vi "Read Configuration.vi"(8 "error in (no error)":errorcluster, 11 "Measure Object in":refnum<class "da Base.lvclass">) -> (0 "error out":errorcluster, 2 "Configuration":variant, 3 "Measure Object out":refnum<class "da Base.lvclass">)   [LabVIEW 2016, in "da Base.lvclass"]
uses:
  da Base.lvclass
  da Base.lvclass/da Base.ctl
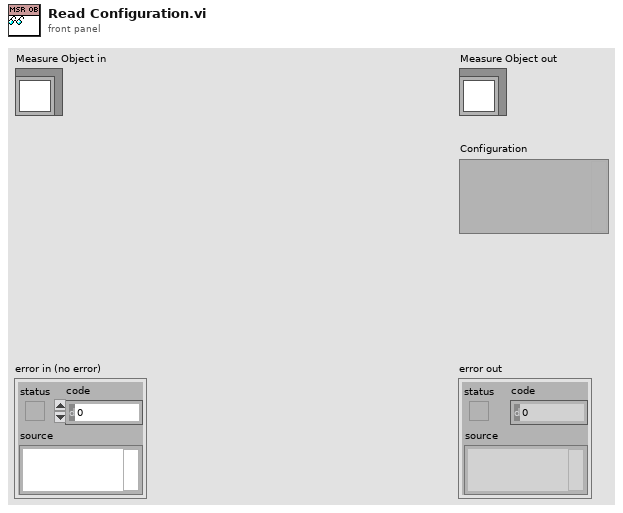
[diagram p1: front panel]
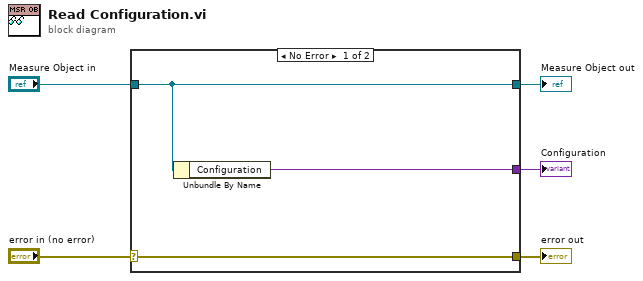
[diagram p0: block diagram]
diagram:
  n1 = case shown="No Error" "error in (no error)" {
    selector: "error in (no error)" -> [w8 w9]
    tunnel: [w8 w9] -> w4
    tunnel: [w7 w10] -> w2
    tunnel: "Measure Object in" -> [w7 w10]
    tunnel: [w6 _] -> w1
    frame No Error {
      n2 = Unbundle By Name(w7) -> ("Configuration"=w6:variant)
    }
    frame Error {
    }
  }
  "error out" <- w4
  "Measure Object out" <- w2
  "Configuration" <- w1
